vi "lectura_config_env.vi"(0 "COM Bluegiga in":refnum<visa-resource-name>, 3 "Handle table":string[][](array[string]), 7 "error in (no error)":errorcluster, 12 "Service UUID":string, 13 "Connection Status":T1={"MAC Address"="", "cnx handle"=0, "cnx flags"=0, "Address Type"=125, "Connection Interval (ms)"=125, "Timeout(ms)"=125, "Latency"=0, "bonding handle"=0} {"Address Type" items=["Public", "Random"]}, 14 "Characteristic UUID":string) -> (15 "COM Bluegiga out":refnum<visa-resource-name>, 17 "error out":errorcluster, 20 "Red intensity":u8, 21 "Green intensity":u8, 22 "Blue intensity":u8, 23 "Gas mode":u8, 24 "Color interval":u16, 25 "Pressure interval":u16, 26 "Temp interval":u16, 27 "Humidity interval":u16)   [LabVIEW 2020]
uses:
  <vilib>/BLE/type_def/connection_status_bundle.ctl
  <vilib>/BLE/type_def/address_type.ctl
panel:
  out "characteristic value":u8[](array[numeric])
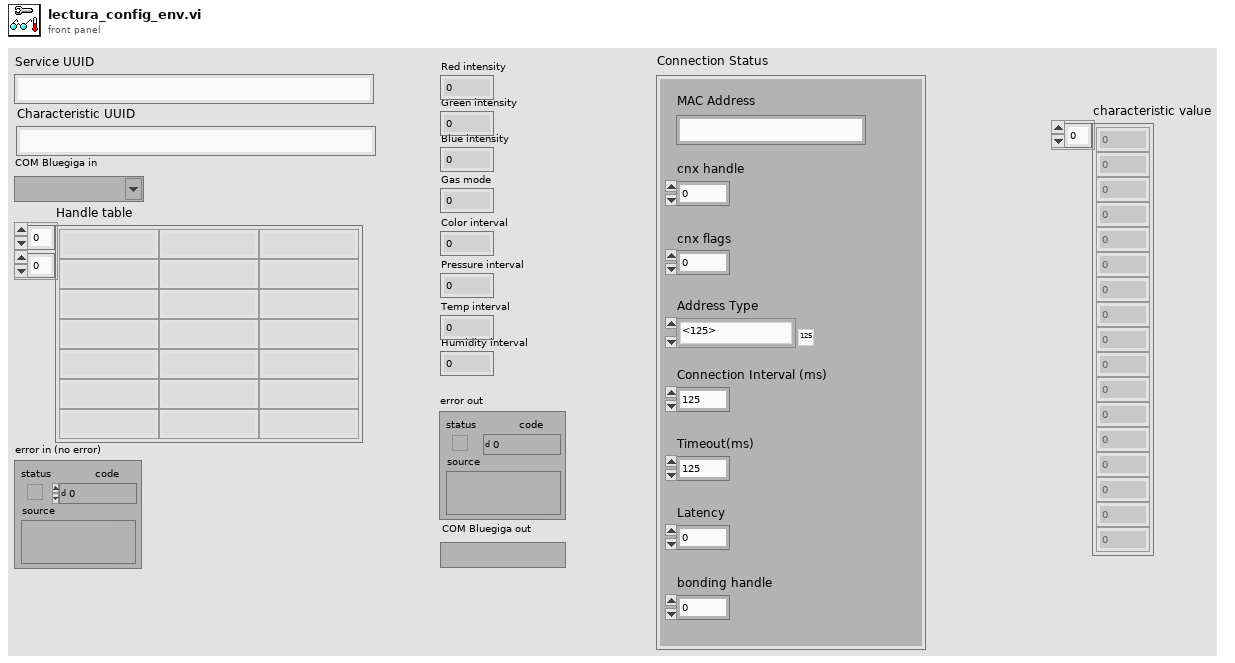
[diagram p1: front panel]
types:
  T1 = typedef "connection_status_bundle.ctl" = cluster{"MAC Address":string, "cnx handle":u8, "cnx flags":u8, "Address Type":T2, "Connection Interval (ms)":u16, "Timeout(ms)":u16, "Latency":u16, "bonding handle":u8}
  T2 = typedef "address_type.ctl" = u8
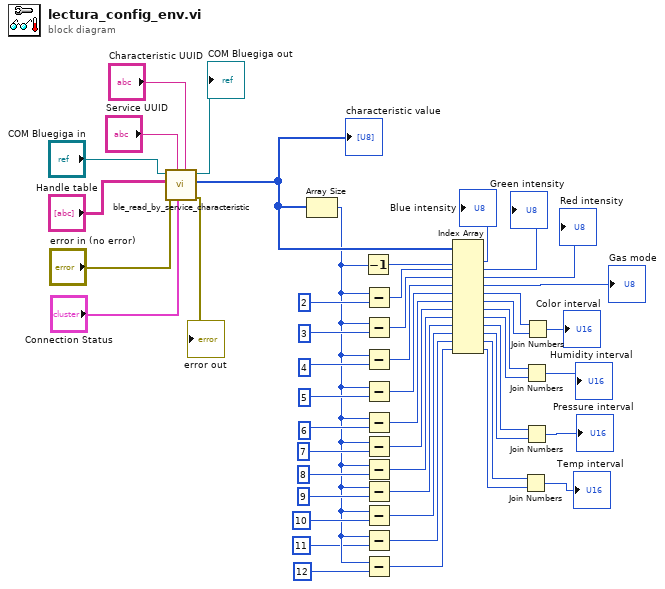
[diagram p0: block diagram]
diagram:
  n1 = call <vilib>:"ble_read_by_service_characteristic.vi"("Characteristic UUID"="Characteristic UUID", "Connection Status"="Connection Status", "Service UUID"="Service UUID", "error in (no error)"="error in (no error)", "Handle table"="Handle table", "COM Bluegiga in"="COM Bluegiga in") -> ("error out"=→"error out":errorcluster, "characteristic value"=w41:u8[], "COM Bluegiga out"=→"COM Bluegiga out":refnum<visa-resource-name>)  [unwired: 3 in]
  "characteristic value" <- w41
  n2 = Array Size(array=w41) -> (size(s)=w10:i32)
  n3 = Decrement(x=w10) -> (x-1=w40:i32)
  n4 = Subtract(x=w10, y=2) -> (x-y=w33:i32)
  n5 = Subtract(x=w10, y=3) -> (x-y=w32:i32)
  n6 = Subtract(x=w10, y=4) -> (x-y=w31:i32)
  n7 = Subtract(x=w10, y=5) -> (x-y=w30:i32)
  n8 = Subtract(x=w10, y=6) -> (x-y=w29:i32)
  n9 = Subtract(x=w10, y=7) -> (x-y=w18:i32)
  n10 = Subtract(x=w10, y=8) -> (x-y=w17:i32)
  n11 = Subtract(x=w10, y=9) -> (x-y=w16:i32)
  n12 = Subtract(x=w10, y=10) -> (x-y=w15:i32)
  n13 = Subtract(x=w10, y=11) -> (x-y=w7:i32)
  n14 = Subtract(x=w10, y=12) -> (x-y=w6:i32)
  n15 = Index Array(array=w41, index #1=w40, index #2=w33, index #3=w32, index #4=w31, index #5=w30, index #6=w29, index #7=w18, index #8=w17, index #9=w16, index #10=w15, index #11=w7, index #12=w6) -> (element #1=→"Blue intensity":u8, element #2=→"Green intensity":u8, element #3=→"Red intensity":u8, element #4=→"Gas mode":u8, element #5=w25:u8, element #6=w24:u8, element #7=w14:u8, element #8=w13:u8, element #9=w12:u8, element #10=w11:u8, element #11=w3:u8, element #12=w2:u8)
  n16 = Join Numbers(hi=w3, lo=w2) -> ((hi.lo)=→"Temp interval":u16)
  n17 = Join Numbers(hi=w14, lo=w13) -> ((hi.lo)=→"Humidity interval":u16)
  n18 = Join Numbers(hi=w12, lo=w11) -> ((hi.lo)=→"Pressure interval":u16)
  n19 = Join Numbers(hi=w25, lo=w24) -> ((hi.lo)=→"Color interval":u16)
